vi "Arrays 1.vi"() -> ()   [LabVIEW 2022 SP3]
panel:
  out "appended array":dbl[](array[numeric])
  in  "Tank 3":dbl(slide) scale=0.0..10.0
  in  "Tank 2":dbl(slide) scale=0.0..10.0
  in  "Tank":dbl(slide) scale=0.0..10.0
  in  "dimension size":i32
  out "initialized array":dbl[](array[numeric])
  out "deleted portion":dbl[](array[numeric])
  out "array w/ subset deleted":dbl[](array[numeric])
  in  "Array 3":dbl[](array[knob]) scale=0.0..10.0
  out "Porcion de array 2 de \narray eliminado":dbl[](array[numeric])
  out "Resultado del \ndelete del array 2":dbl[](array[numeric])
  out "Array  con elemento \n15 insertado":dbl[](array[numeric])
  in  "Gauge":dbl(knob) scale=0.0..10.0
  out "Array dbl con elemeto r30 remplazado en la posicion 1 y 0 con un gauge":dbl[](array[numeric])
  out "size(s) 2":i32
  in  "Array 2":dbl[](array[numeric])
  out "3":string
  out "2":string
  in  "control":i32
  out "1":string
  out "size(s)":i32
  in  "Array":string[](array[string])
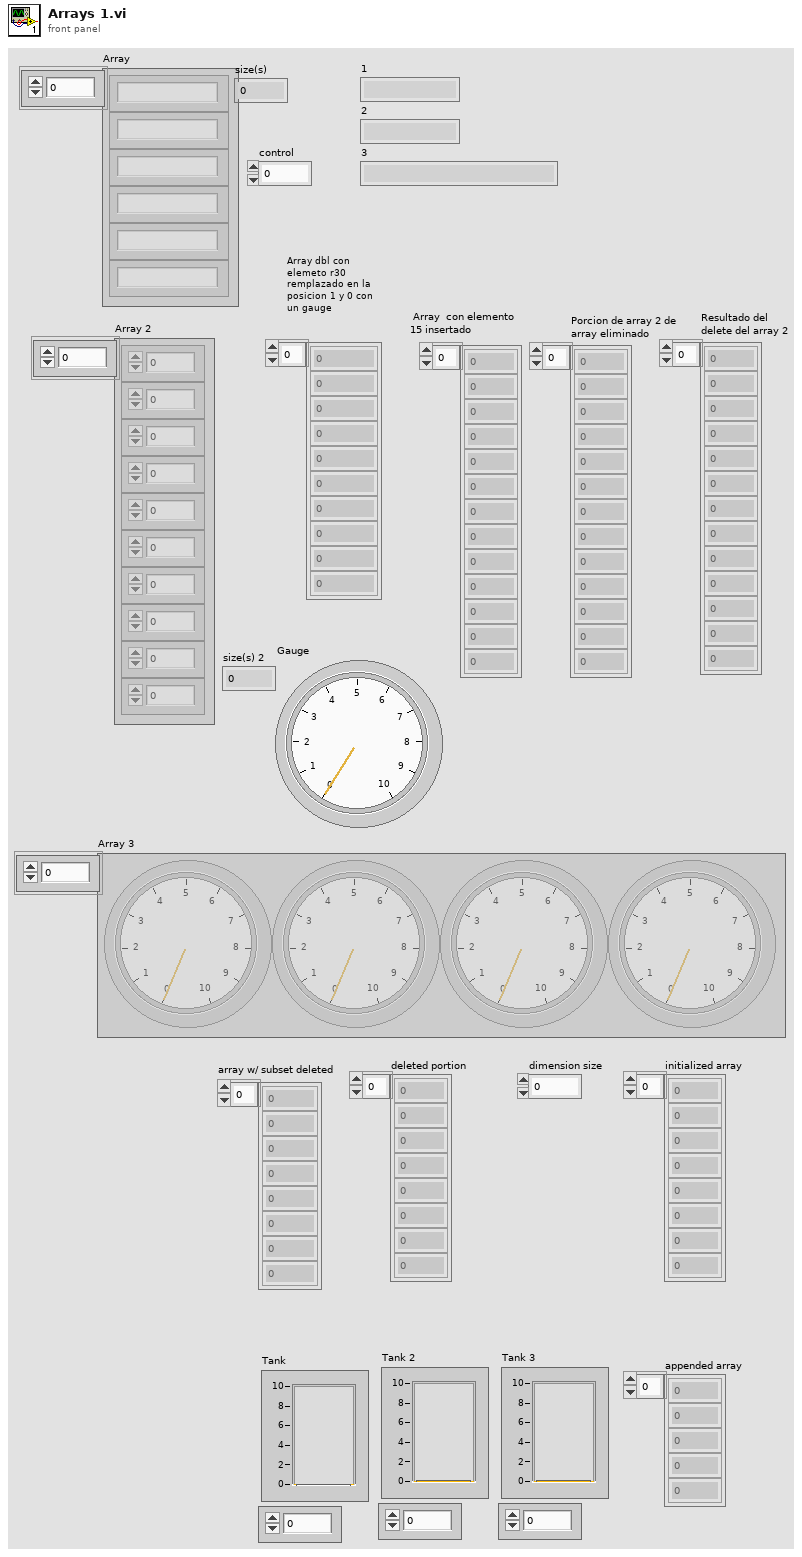
[diagram p1: front panel]
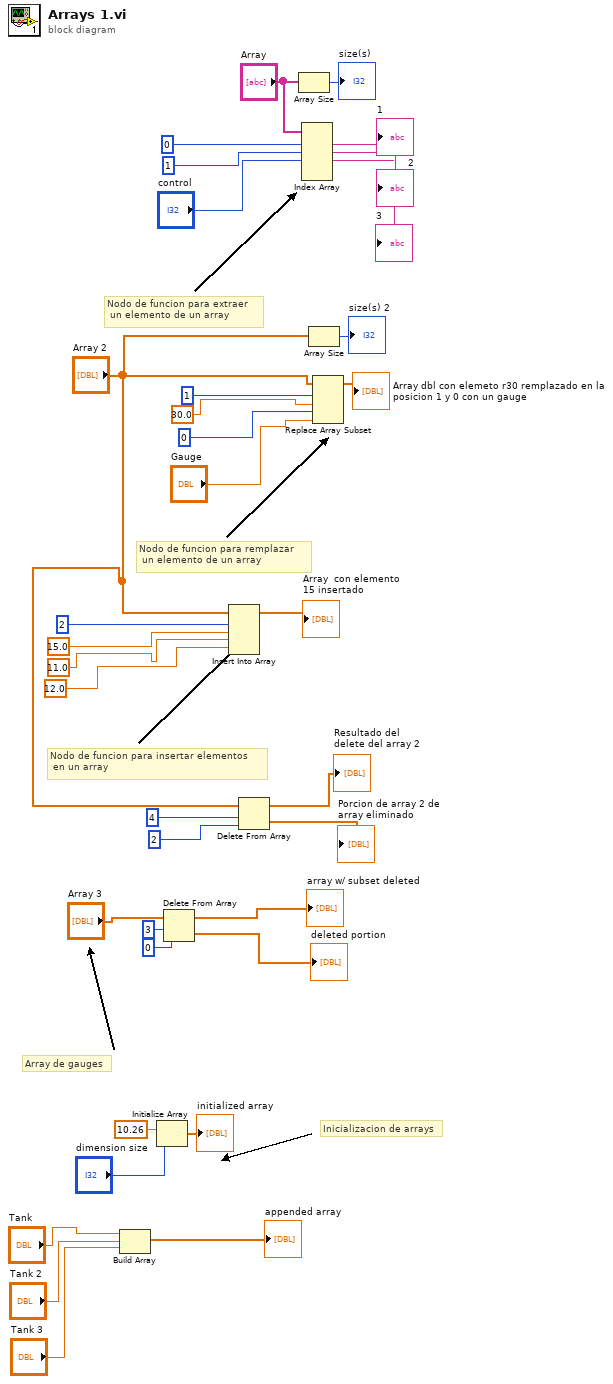
[diagram p0: block diagram]
diagram:
  # "Inicializacion de arrays"
  # "Array de gauges"
  # "Nodo de funcion para insertar elementos\n en un array"
  # "Nodo de funcion para remplazar\n un elemento de un array"
  # "Nodo de funcion para extraer\n un elemento de un array"
  n1 = Build Array("Tank", "Tank 2", "Tank 3") -> (→"appended array":dbl[])
  n2 = Initialize Array(10.26 ("element"), "dimension size") -> (→"initialized array":dbl[])
  n3 = Delete From Array(array="Array 3", length=3, index=0) -> (deleted portion=→"deleted portion":dbl[], array with subset deleted=→"array w/ subset deleted":dbl[])
  n4 = Insert Into Array(array="Array 2", index=2, new element #1=15.0 ("new element/subarray"), new element #2=11.0 ("new element/subarray"), new element #3=12.0 ("new element/subarray")) -> (→"Array  con elemento \n15 insertado":dbl[])
  n5 = Delete From Array(array="Array 2", length=4, index=2) -> (deleted portion=→"Porcion de array 2 de \narray eliminado":dbl[], array with subset deleted=→"Resultado del \ndelete del array 2":dbl[])
  n6 = Array Size(array="Array") -> (size(s)=→"size(s)":i32)
  n7 = Index Array(array="Array", index #1=0 ("index"), index #2=1 ("index"), index #3="control") -> (element #1=→"1":string, element #2=→"2":string, element #3=→"3":string)  [unwired: 2 in, 2 out]
  n8 = Array Size(array="Array 2") -> (size(s)=→"size(s) 2":i32)
  n9 = Replace Array Subset(array="Array 2", new element #1=30.0 ("new element/subarray"), index #1=1 ("index"), new element #2="Gauge", index #2=0 ("index")) -> (→"Array dbl con elemeto r30 remplazado en la posicion 1 y 0 con un gauge":dbl[])
